vi "WriteWAVFile.vi"(8 "error in (no error)":errorcluster, 10 "Waveform":waveform(dbl), 11 "Path":path) -> (0 "error out":errorcluster)   [LabVIEW 2017]
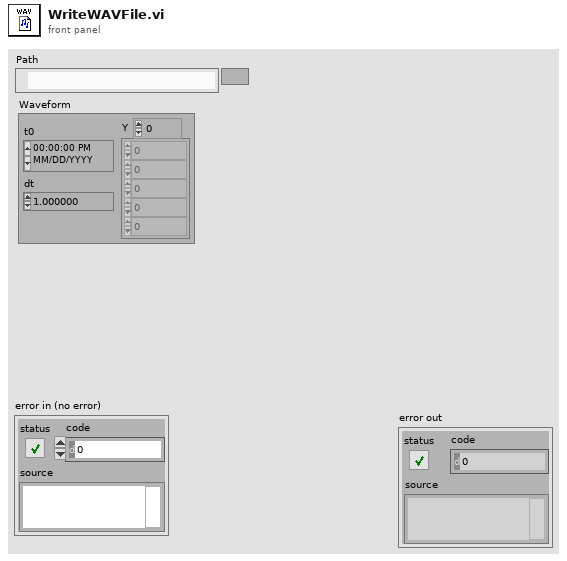
[diagram p1: front panel]
types:
  T1 = enum16{"open", "replace", "create", "open or create", "replace or create", "replace or create with confirmation"}
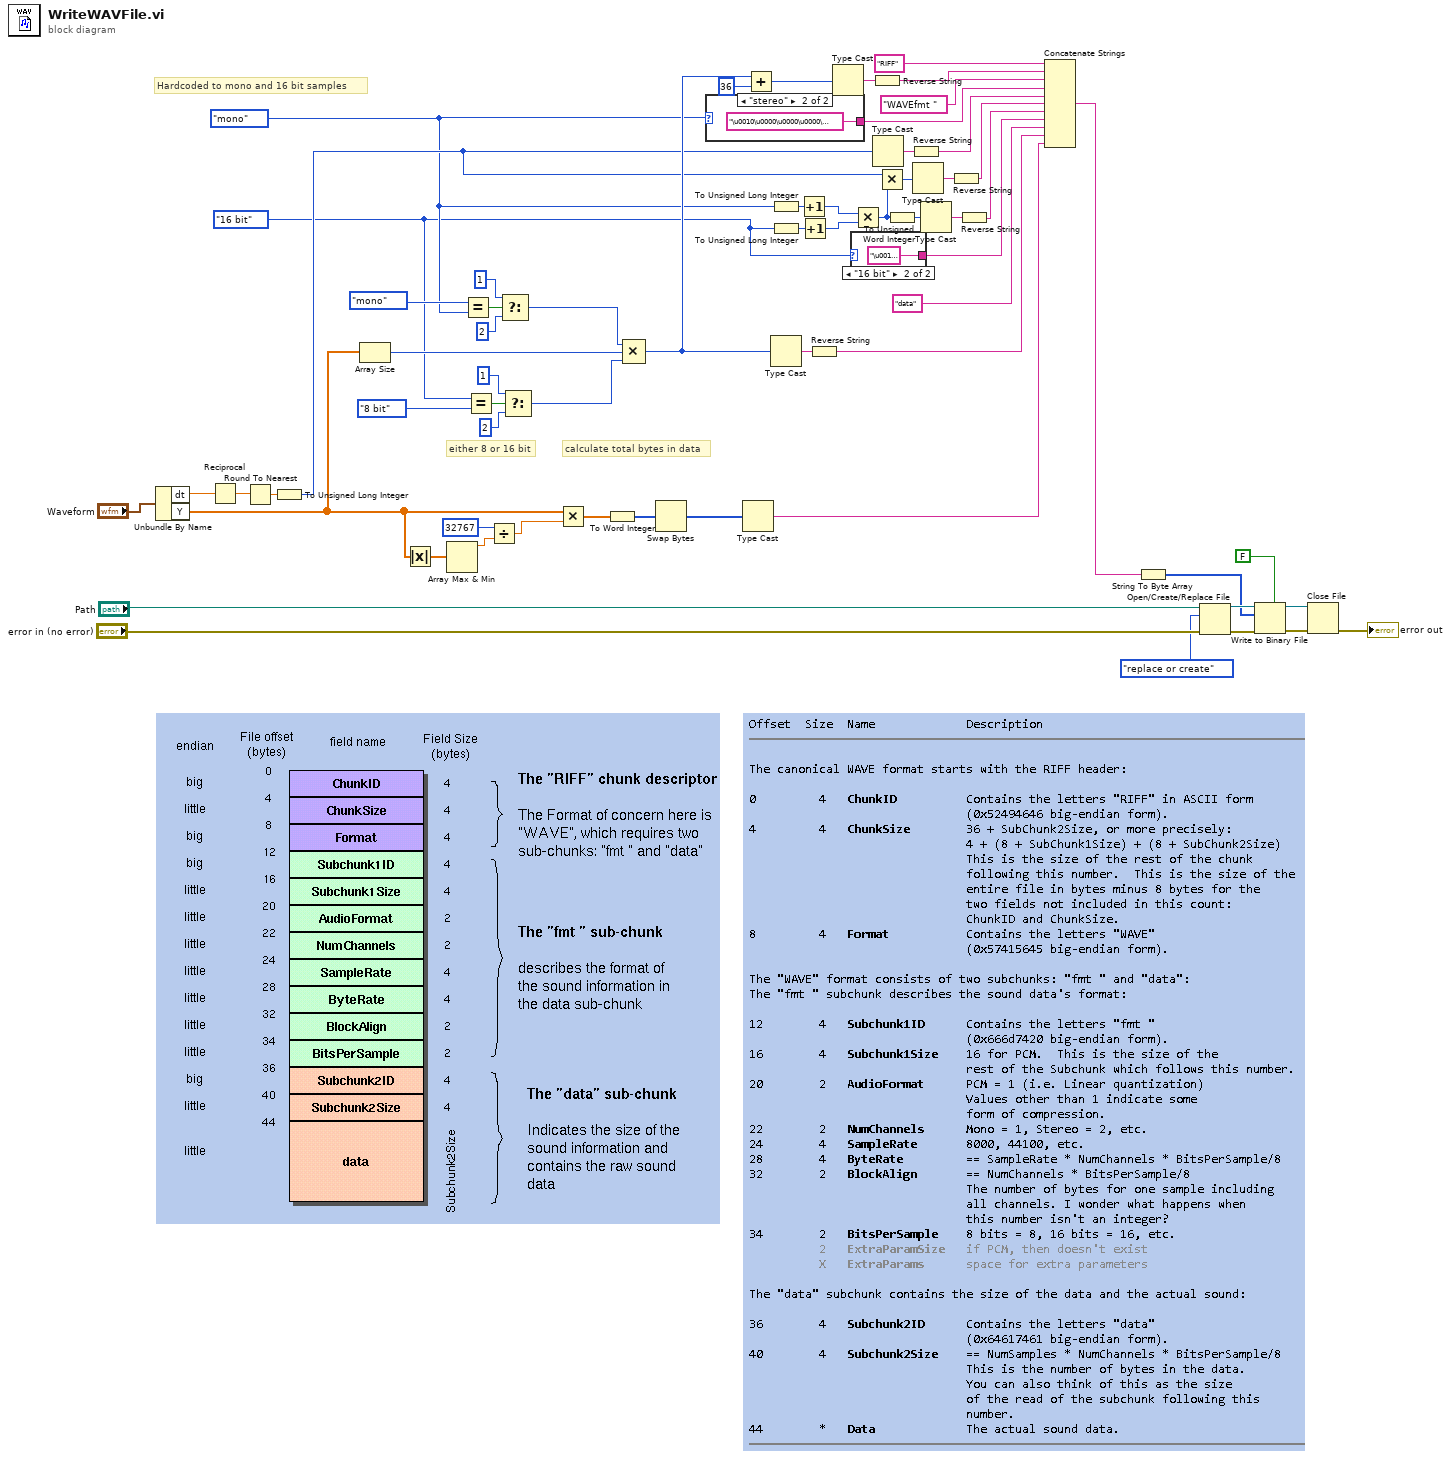
[diagram p0: block diagram]
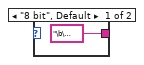
[diagram p2: hidden frame]
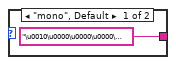
[diagram p3: hidden frame]
diagram:
  w1 = enum16{"8 bit", "16 bit"}."16 bit" ("bits per sample")
  w2 = enum16{"mono", "stereo"}."mono" ("sound quality")
  # "Hardcoded to mono and 16 bit samples"
  # "calculate total bytes in data"
  # "either 8 or 16 bit"
  n1 = Unbundle By Name("Waveform") -> ("dt"=w6:dbl, "Y"=w21:dbl[])
  n2 = Reciprocal(x=w6) -> (1/x=w5:dbl)
  n3 = Round To Nearest(number=w5) -> (nearest integer value=w4:dbl)
  n4 = To Unsigned Long Integer(number=w4) -> (unsigned 32bit integer=w3:u32)
  n5 = Array Size(array=w21) -> (size(s)=w29:i32)
  n6 = Absolute Value(x=w21) -> (abs(x)=w26:dbl[])
  n7 = Array Max & Min(array=w26) -> (max value=w24:dbl)  [unwired: 3 out]
  n8 = Equal?(x=enum16{"mono", "stereo"}."mono" ("sound quality"), y=w2) -> (x = y?=w40:bool)
  n9 = Equal?(x=w1, y=enum16{"8 bit", "16 bit"}."8 bit") -> (x = y?=w36:bool)
  n10 = Divide(x=i16 32767, y=w24) -> (x/y=w23:dbl)
  n11 = Select(t=1, s=w40, f=2) -> (s? t:f=w37:i32)
  n12 = Select(t=1, s=w36, f=2) -> (s? t:f=w32:i32)
  n13 = Multiply(x=w21, y=w23) -> (x*y=w22:dbl[])
  n14 = To Word Integer(number=w22) -> (16bit integer=w28:i16[])
  n15 = Compound Arithmetic op=MULTIPLY(w37, w29, w32) -> (w31:i32)
  n16 = Swap Bytes(anything=w28) -> (byte swapped=w27:i16[])
  n17 = case shown="\"stereo\"" w2 {
    tunnel: ["\u0010\u0000\u0000\u0000\u0001\u0000\u0001\u0000" "\u0010\u0000\u0000\u0000\u0001\u0000\u0002\u0000"] -> w43
    frame "mono", Default {
    }
    frame "stereo" {
    }
  }
  n18 = Type Cast(x=w27) -> (*(type *) &x=w8:string)  [unwired: 1 in]
  n19 = Add(x=w31, y=36) -> (x+y=w7:i32)
  n20 = To Unsigned Long Integer(number=w2) -> (unsigned 32bit integer=w52:u32)
  n21 = To Unsigned Long Integer(number=w1) -> (unsigned 32bit integer=w51:u32)
  n22 = Type Cast(x=w31) -> (*(type *) &x=w61:string)  [unwired: 1 in]
  n23 = Increment(x=w52) -> (x+1=w50:u32)
  n24 = Increment(x=w51) -> (x+1=w49:u32)
  n25 = Reverse String(1:w61) -> (0:w44:string)
  n26 = Type Cast(x=w7) -> (*(type *) &x=w60:string)  [unwired: 1 in]
  n27 = case shown="\"16 bit\"" w1 {
    tunnel: ["\b\u0000" "\u0010\u0000"] -> w42
    frame "8 bit", Default {
    }
    frame "16 bit" {
    }
  }
  n28 = Multiply(x=w50, y=w49) -> (x*y=w47:u32)
  n29 = Reverse String(1:w60) -> (0:w58:string)
  n30 = Type Cast(x=w3) -> (*(type *) &x=w57:string)  [unwired: 1 in]
  n31 = Multiply(x=w3, y=w47) -> (x*y=w53:u32)
  n32 = To Unsigned Word Integer(number=w47) -> (unsigned 16bit integer=w46:u16)
  n33 = Reverse String(1:w57) -> (0:w56:string)
  n34 = Type Cast(x=w53) -> (*(type *) &x=w55:string)  [unwired: 1 in]
  n35 = Type Cast(x=w46) -> (*(type *) &x=w48:string)  [unwired: 1 in]
  n36 = Reverse String(1:w55) -> (0:w54:string)
  n37 = Reverse String(1:w48) -> (0:w45:string)
  n38 = Concatenate Strings("RIFF", w58, "WAVEfmt ", w43, w56, w54, w45, w42, "data", w44, w8) -> (w11:string)
  n39 = String To Byte Array(string=w11) -> (unsigned byte array=w10:u8[])
  n40 = Open/Create/Replace File(file path (use dialog)="Path", error in="error in (no error)", operation (0:open)=T1."replace or create") -> (refnum out=w17:refnum<file>, error out=w18:errorcluster)  [unwired: 3 in, 1 out]
  n41 = Write to Binary File(file (use dialog)=w17, data=w10, error in=w18, 5:FALSE ("prepend array or string size? (T)")) -> (refnum out=w15:refnum<file>, error out=w16:errorcluster)  [unwired: 2 in, 1 out]
  n42 = Close File(refnum=w15, error in=w16) -> (error out=→"error out":errorcluster)  [unwired: 1 out]
